vi "Dashboard Main.vi"() -> ()   [LabVIEW 2012]
uses:
  2013ROBOT!/Auto State Selector.ctl
  <vilib>/event_ctls.llb/eventvkey.ctl
  <vilib>/Utility/config.llb/Read Key (String).vi
  <vilib>/Utility/config.llb/Read Key (I32).vi
  <vilib>/Utility/config.llb/Write Key (String).vi
  <vilib>/Utility/config.llb/Write Key (I32).vi
  <vilib>/Utility/config.llb/NI_LVConfig.lvlib
panel:
  out "Bail Climb":bool
  out "Big Hooks on Bar":bool
  out "High gear - Low gear":bool
  out "Shooter Speed (ft/s)":dbl(knob) scale=0.0..400.0
  in  "Auto State Selector":T1
  out "Battery?":u8(slide) scale=0.0..100.0
  out "Tank Pressure (psi)":dbl(knob) scale=0.0..200.0
  out "Compressor":bool
  out "Climbing":bool
  in  "Camera Settings":T2={"Frate Rate"=30, "Compression"=30, "Size"=1} {"Frate Rate" scale=1.0..30.0; "Size" items=["640x480", "320x240", "160x120"]}
  out "Mode":T3(ring)=enum."Auto Disabled"
  out "Camera IP":string
  out "Robot IP":string
  in  "Dashboard Tab":enum32{"Operation", "Test", "Checklist"}(tab)
  in  "Slider":dbl(slide) scale=0.0..100.0 scale format="%#_3g"
  in  "On/Off":bool caption="Solenoid"
  in  "Test Name":u16(ring) items=["Select the test to run...", "Example Test", "-------------------------------", "List of tests is built in robot code.", "Replace with your own automated tests."]
  in  "Test Tree":string(tree)
  in  "Motor":cluster{"Value":dbl, "Enable":bool} {"Value" scale=-1.0..1.0 scale format="%#_3g"}
  out "Progress":T4 {"Test Progress" scale=0.0..100.0}
  in  "Rev/Fwd":cluster{"Forward":bool, "Reverse":bool}
  in  "Ring":u16(ring) items=["Auto", "Fixed indoor", "Fixed outdoor 1", "Fixed outdoor 2", "Fixed fluorescent 1", "Fixed fluorescent 2", "Hold current"]
  in  "Listbox":i32(listbox)
  in  "Viewer":T5(tab)
  out "Mbps":dbl format="%#.1g"
  in  "Enable":bool
  in  "DB Camera Config":bool
  out "Mbps":bool
  out "fps":dbl format="%#.1g"
  out "Image Error Message":string="Timeout in Camera Communications"
  out "Camera Image":T6(plugin-control)
  out "Autolock":bool
  out "Distance from goal (ft)":dbl(slide) scale=0.0..30.0
  out "Buttons 1":cluster{"1":bool, "2":bool, "3":bool}
  out "Kinect 1":cluster{"X":dbl, "Y":dbl, "Z":dbl} {"X" scale=1.0..-1.0; "Y" scale=1.0..-1.0; "Z" scale=1.0..-1.0}
  out "Buttons 2":cluster{"1":bool, "2":bool, "3":bool}
  out "Kinect 2":cluster{"X":dbl, "Y":dbl, "Z":dbl} {"X" scale=1.0..-1.0; "Y" scale=1.0..-1.0; "Z" scale=1.0..-1.0}
  out "Version":string
  out "Skeleton Picture":picture
  out "Players":i8
  out "Tree":string(tree)
  # "Robot IP:"
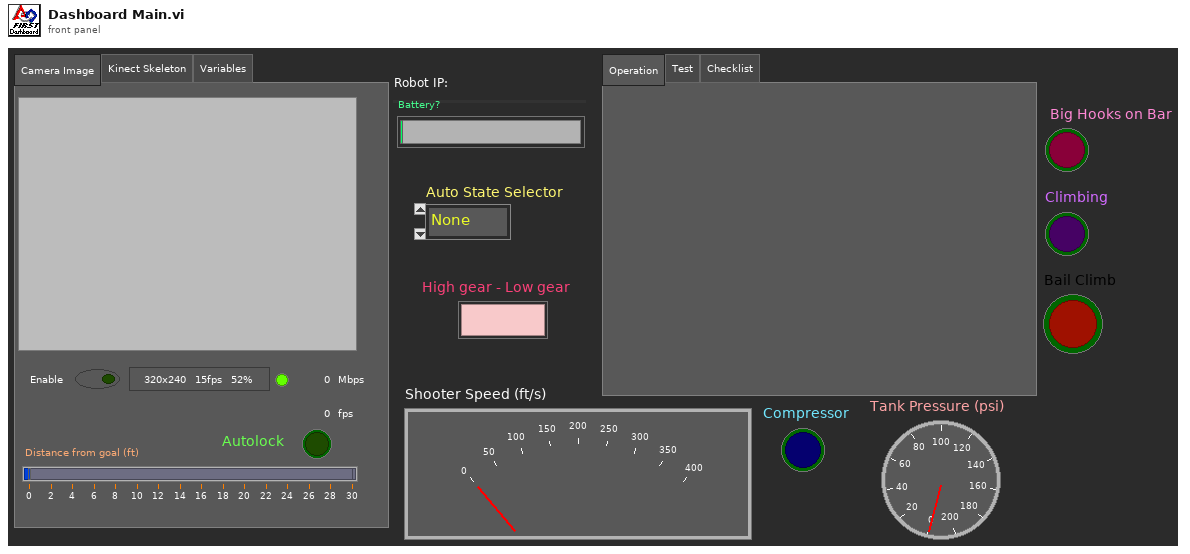
[diagram p1: front panel]
types:
  T1 = typedef "Auto State Selector.ctl" = enum16{"None", "Fire 2x", "Fire 3x", "Dump in low goal"}
  T2 = cluster{"Frate Rate":i32, "Compression":i32, "Size":u16}
  T3 = enum8{"Tele-Op Disabled", "Tele-Op Enabled", "Auto Disabled", "Auto Enabled", "Test Disabled", "Test Enabled", ""}
  T4 = cluster{"Test Progress":u8, "Test Progress Text":string}
  T5 = enum32{"Camera Image", "Kinect Skeleton", "Variables"}
  T6 = typedef "IMAQ Image.ctl" = refnum<image>
  T7 = typedef "Image Type" = u32
  T8 = typedef "LVBoundsTypeDef.ctl" = cluster{"Width":u32, "Height":u32}
  T9 = typedef "SkeletonTrackState.ctl" = enum32{"NotTracked", "PositionOnly", "Tracked"}
  T10 = cluster{"TrackingState":u8[], "Position":cluster{"x":sgl, "y":sgl, "z":sgl}, cluster{"x":sgl, "y":sgl, "z":sgl, sgl}[], "TrackState":T9}
  T11 = cluster{cluster{"ScaledToPercentRange":dbl, "ScaledToPercentRange":dbl, "ScaledToPercentRange":dbl}, cluster{bool, bool, bool}}[]
  T12 = cluster{cluster{"ScaledToPercentRange":dbl, "ScaledToPercentRange":dbl, "ScaledToPercentRange":dbl}, cluster{bool, bool, bool}}
  T13 = cluster{"ScaledToPercentRange":dbl, "ScaledToPercentRange":dbl, "ScaledToPercentRange":dbl}
  T14 = typedef "LVRectTypeDef.ctl" = cluster{"Left":i16, "Top":i16, "Right":i16, "Bottom":i16}
  T15 = cluster{"Competition mode":bool, "Robot Link":bool, "Autonomous":bool, "Enabled":bool, "E-Stop":bool, "Simulated":bool, "TestMode":bool, "Docked Window":bool}
  T16 = typedef "NI_LVConfig.lvlib/Config Data RefNum.ctl" = refnum<k1>
  T17 = typedef "eventvkey.ctl" = enum16{"ASCII", "Enter", "Return", "Shift", "Ctrl", "Alt", "Cmd", "Opt", "Caps", "NumLock", "Clear", "Break", "Up", "Down", "Left", "Right", "Insert", "Delete", "Home", "End", "PageUp", "PageDown", "Escape", "Help", "Pause", "ScrollLock", "F1", "F2", "F3", "F4", "F5", "F6", "F7", "F8", "F9", "F10", "F11", "F12", "F13", "F14", "F15", "F16", "F17", "F18", "F19", "F20", "F21", "F22", "F23", "F24", "Play", "VolumeUp", "VolumeDown", "Mute", "Two Byte Char"}
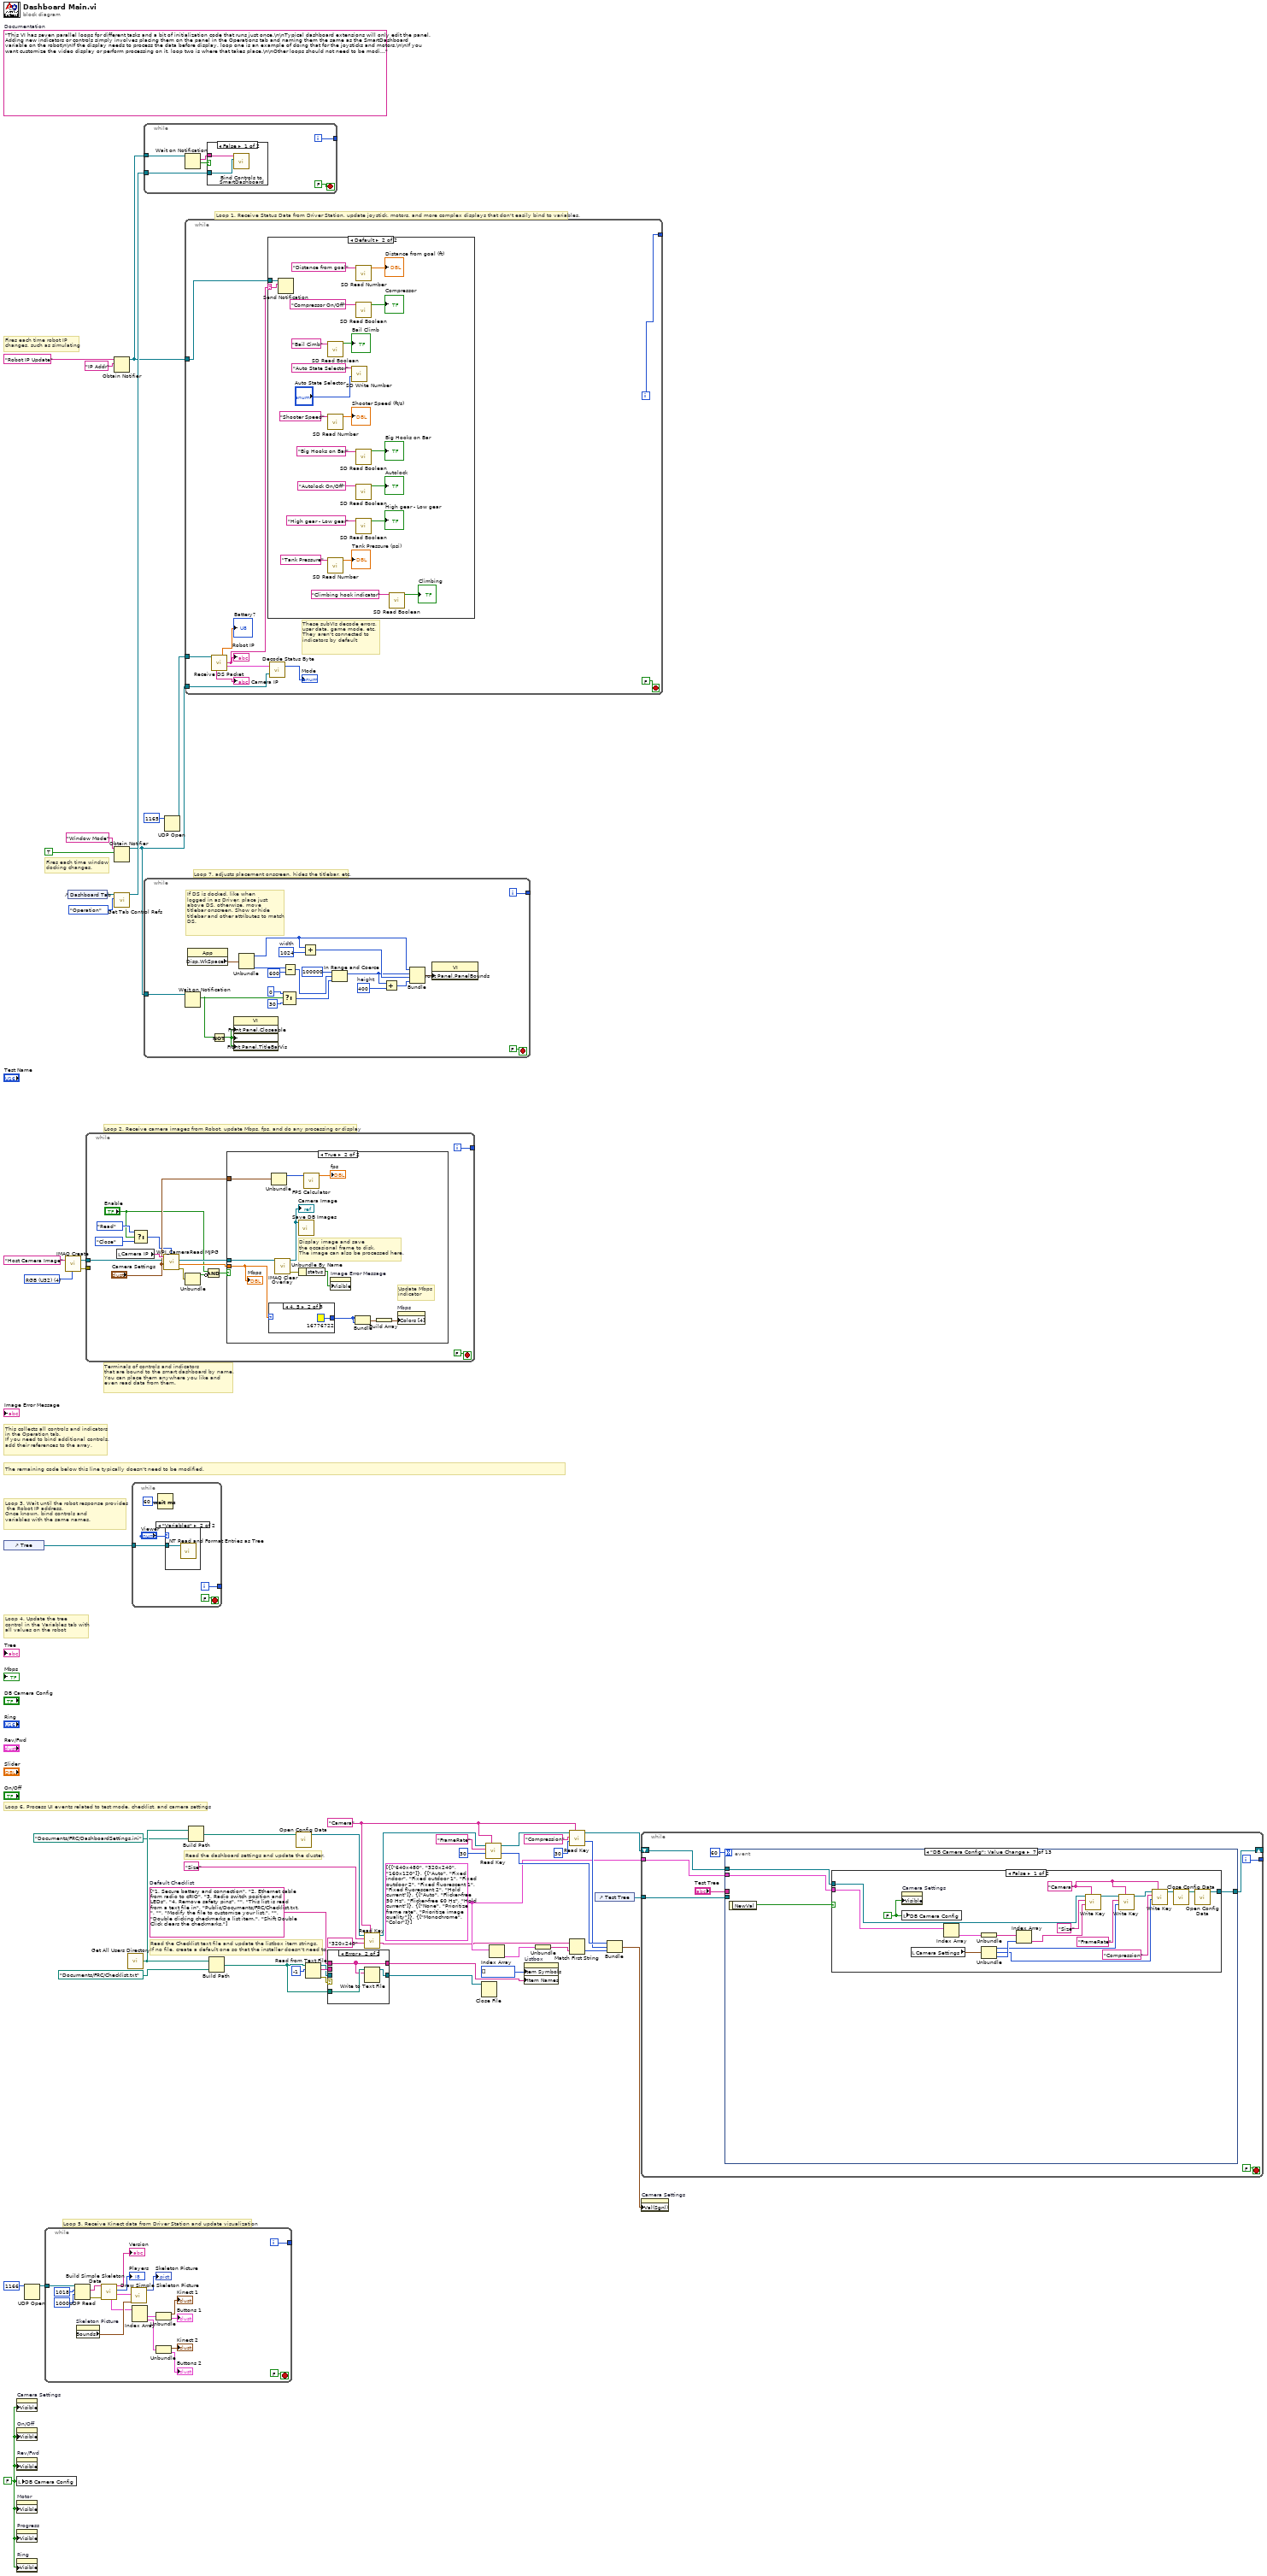
[diagram p0: block diagram]
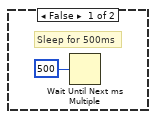
[diagram p3: hidden frame]
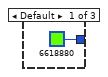
[diagram p4: hidden frame]
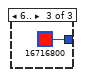
[diagram p5: hidden frame]
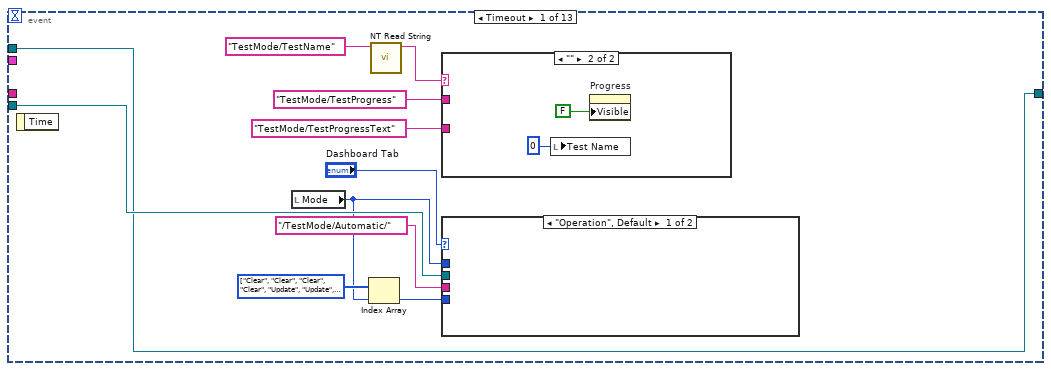
[diagram p7: hidden frame]
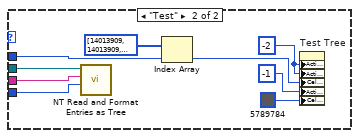
[diagram p8: hidden frame]
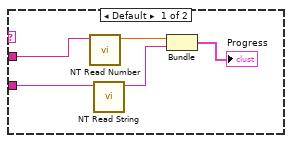
[diagram p9: hidden frame]
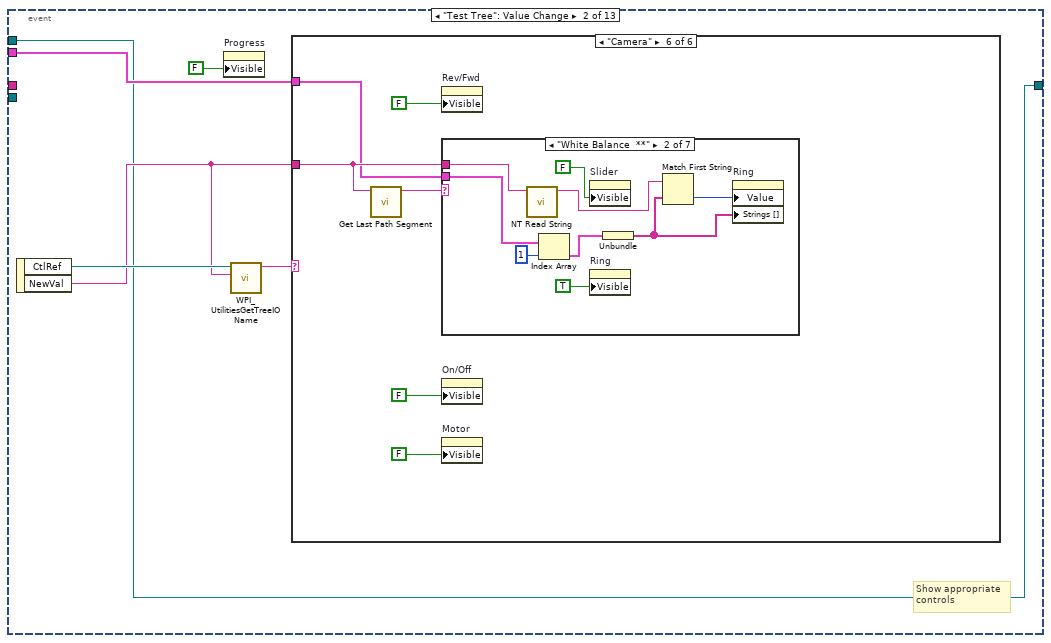
[diagram p10: hidden frame]
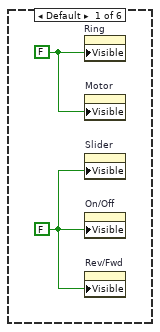
[diagram p11: hidden frame]
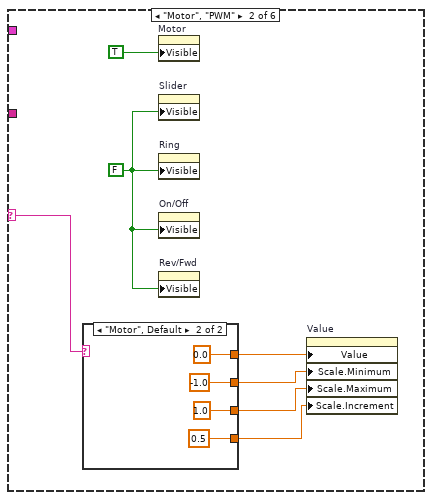
[diagram p12: hidden frame]
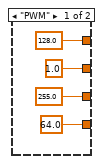
[diagram p13: hidden frame]
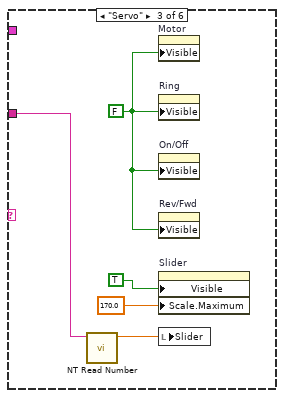
[diagram p14: hidden frame]
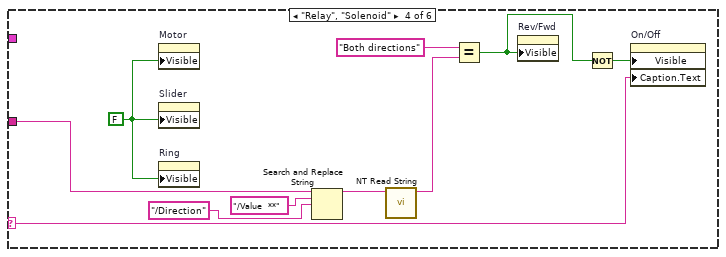
[diagram p15: hidden frame]
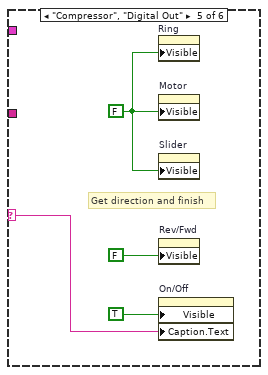
[diagram p16: hidden frame]
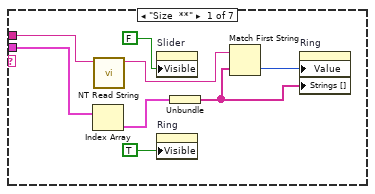
[diagram p17: hidden frame]
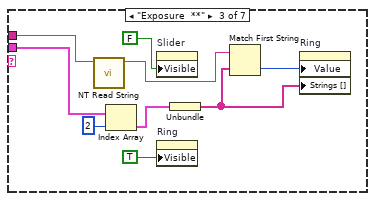
[diagram p18: hidden frame]
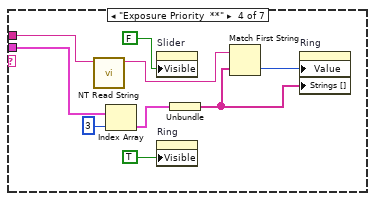
[diagram p19: hidden frame]
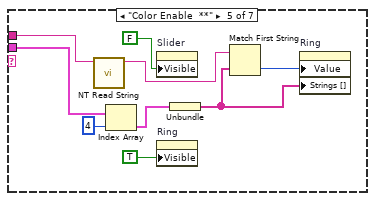
[diagram p20: hidden frame]
diagram:
  w21 = "Camera"
  w13 = cluster{string[]}[] [{["640x480", "320x240", "160x120"]}, {["Auto", "Fixed indoor", "Fixed outdoor 1", "Fixed outdoor 2", "Fixed fluorescent 1", "Fixed fluorescent 2", "Hold current"]}, {["Auto", "Flicker-free 50 Hz", "Flicker-free 60 Hz", "Hold current"]}, {["None", "Prioritize frame rate", "Prioritize image quality"]}, {["Monochrome", "Color"]}]
  w29 = string[] ["1. Secure battery and connection", "2. Ethernet cable from radio to cRIO", "3. Radio switch position and LEDs", "4. Remove safety pins", "", "This list is read from a text file in", "Public/Documents/FRC/Checklist.txt.", "", "Modify the file to customize your list.", "", "Double clicking checkmarks a list item.", "Shift Double Click clears the checkmarks."]  # Default Checklist
  w27 = FALSE ("Visible")
  (unwired) "This VI has seven parallel loops for different tasks and a bit of initialization code that runs just once.\n\nTypical dashboard extensions will only edit the panel. Adding new indicators or controls simply involves placing them on the panel in the Operations tab and naming them the same as the SmartDashboard variable on the robot\n\nIf the display needs to process the data before display, loop one is an example of doing that for the joysticks and motors.\n\nIf you want customize the video display or perform processing on it, loop two is where that takes place.\n\nOther loops should not need to be modified. They are pretty standard, and document the task they perform."  # Documentation
  w50 = T7 4 items=["Grayscale (U8)", "Grayscale (I16)", "Grayscale (SGL)", "Complex (CSG)", "RGB (U32)", "HSL (U32)", "RGB (U64)"] ("Image Type")
  # "Fires each time robot IP\nchanges, such as simulating"
  # "Fires each time window\ndocking changes."
  # "Read the Checklist text file and update the listbox item strings.\nIf no file, create a default one so that the installer doesn't need to."
  # "This collects all controls and indicators\nin the Operation tab.\nIf you need to bind additional controls,\nadd their references to the array."
  # "The remaining code below this line typically doesn't need to be modified."
  # "Loop 6. Process UI events related to test mode, checklist, and camera settings"
  # "Read the dashboard settings and update the cluster."
  # "Terminals of controls and indicators\nthat are bound to the smart dashboard by name.\nYou can place them anywhere you like and\neven read data from them."
  # "Loop 4. Update the tree\ncontrol in the Variables tab with\nall values on the robot"
  # "Loop 3. Wait until the robot response provides\n the Robot IP address.\nOnce known, bind controls and\nvariables with the same names."
  # "Loop 5. Receive Kinect data from Driver Station and update visualization"
  # "Loop 7. adjusts placement onscreen, hides the titlebar, etc."
  # "Loop 1. Receive Status Data from Driver Station, update joystick, motors, and more complex displays that don't easily bind to variables."
  # "Loop 2. Receive camera images from Robot, update Mbps, fps, and do any processing or display"
  n1 = control-ref of="Tree"() -> (w2:refnum<vi>)
  n2 = property on="Camera Settings" class="Clust (strict)"("Visible"=w27) -> ()  [unwired: 2 in, 2 out]
  n3 = property on="On/Off" class="Bool (strict)"("Visible"=w27) -> ()  [unwired: 2 in, 2 out]
  n4 = property on="Rev/Fwd" class="Clust (strict)"("Visible"=w27) -> ()  [unwired: 2 in, 2 out]
  n5 = local write "DB Camera Config"(w27) -> ()
  n6 = property on="Motor" class="Clust (strict)"("Visible"=w27) -> ()  [unwired: 2 in, 2 out]
  n7 = property on="Progress" class="Clust (strict)"("Visible"=w27) -> ()  [unwired: 2 in, 2 out]
  n8 = property on="Ring" class="Ring (strict)"("Visible"=w27) -> ()  [unwired: 2 in, 2 out]
  n9 = UDP Open(11:u16 1166 ("port")) -> (port=w45:refnum<k16>)  [unwired: 2 in, 4 out]
  n10 = while {
    tunnel: w45 -> [w69]
    tunnel: [w54] -> _
    i -> [w54]
    stop <- FALSE stop-if-true
    n11 = UDP Read(connection ID=w69, max size (548)=1018 ("bytes to read"), timeout ms (25000)=1000) -> (data out=w63:string, error out=w53:errorcluster)  [unwired: 1 in, 3 out]
    n12 = property on="Skeleton Picture" class="Pict"() -> ("Bounds"=w65:T8)  [unwired: 2 in, 2 out]
    n13 = call "Build Simple Skeleton Data.vi"("error in (no error)"=w53, "data in"=w63) -> ("Skeleton Data"=w64:T10, "NumPlayers"=→"Players":i8, "Version String"=→"Version":string, "Simple Joystick Info"=w61:T11)  [unwired: 5 in, 1 out]
    n14 = call "Draw Simple Skeleton Picture.vi"("Bounds"=w65, "Simple Skeleton"=w64) -> ("new picture out"=→"Skeleton Picture":picture)  [unwired: 9 in]
    n15 = Index Array(array=w61) -> (element #1=w60:T12, element #2=w59:T12)  [unwired: 2 in]
    n16 = Unbundle(w60) -> (→"Kinect 1":T13, →"Buttons 1":cluster{bool, bool, bool})
    n17 = Unbundle(w59) -> (→"Kinect 2":T13, →"Buttons 2":cluster{bool, bool, bool})
  }
  n18 = call "IMAQ Create"("Image Name"="Host Camera Image", "Image Type"=w50) -> ("New Image"=w48:T6, "error out"=w47:errorcluster)  [unwired: 2 in, 1 out]
  n19 = control-ref of="Dashboard Tab"() -> (w43:refnum<vi>)
  n20 = while {
    tunnel: w48 -> [w81]
    tunnel: w47 -> [_]
    tunnel: [w84] -> _
    i -> [w84]
    stop <- FALSE stop-if-true
    n21 = local read "Camera IP"() -> (w83:string)
    n22 = Select(t=enum16{"Read", "Reopen", "Close"}."Read" ("Operation"), s="Enable", f=enum16{"Read", "Reopen", "Close"}."Close" ("Operation")) -> (s? t:f=w76:enum16{"Read", "Reopen", "Close"})
    n23 = call <vilib>:"WPI_CameraRead MJPG.vi"("Operation"=w76, "Camera Settings"="Camera Settings", "Image"=w81, "address"=w83) -> ("error out"=w75:errorcluster, "Bandwidth (kbps)"=w79:dbl, "Image Out"=w80:T6)  [unwired: 5 in]
    n24 = Unbundle(w75) -> ("status"=w73:bool)  [unwired: 2 out]
    n25 = Compound Arithmetic op=AND("Enable", invert w73) -> (w72:bool)
    n26 = case shown="True" w72 {
      tunnel: "Camera Settings" -> [_ w88]
      tunnel: w80 -> [_ w91]
      tunnel: w79 -> [_ w90]
      frame False {
        # "Sleep for 500ms"
        n27 = Wait Until Next ms Multiple(millisecond multiple=u32 500) -> ()  [unwired: 1 out]
      }
      frame True {
        # "Display image and save\nthe occasional frame to disk.\nThe image can also be processed here."
        # "Update Mbps\nindicator"
        n28 = case shown="4, 5" w90 {
          tunnel: [u32 6618880 ("Color Box") u32 16776722 ("Color Box") u32 16716800 ("Color Box")] -> w92
          frame Default {
          }
          frame 4, 5 {
          }
          frame 6.. {
          }
        }
        n29 = Unbundle(w88) -> ("Frate Rate"=w87:i32)  [unwired: 2 out]
        n30 = call "IMAQ Clear Overlay"("Image"=w91) -> ("error out"=w96:errorcluster, "Image Out"=w95:T6)  [unwired: 2 in, 7 out]
        "Camera Image" <- w95
        n31 = call "Save DB Images.vi"("Image"=w95) -> ()  [unwired: 2 in, 1 out]
        n32 = Unbundle By Name(w96) -> ("status"=w97:bool)
        n33 = call "FPS Calculator.vi"("Average Count"=w87) -> ("fps"=→"fps":dbl)  [unwired: 10 in]
        n34 = property on="Image Error Message" class="Str"("Visible"=w97) -> ()  [unwired: 2 in, 2 out]
        n35 = Bundle("Color Box"=w92, "Color Box"=w92) -> (w94:cluster{"Color Box":u32, "Color Box":u32})  [unwired: 1 out]
        n36 = Build Array(w94) -> (w93:cluster{"Color Box":u32, "Color Box":u32}[])
        n37 = property on="Mbps" class="Bool (strict)"("Colors [4]"=w93) -> ()  [unwired: 2 in, 2 out]
        "Mbps" <- w90
      }
    }
  }
  n38 = Obtain Notifier(name (unnamed)="Robot IP Update", notification data type="IP Addr" ("name (unnamed)")) -> (notifier out=w40:refnum<notifier>)  [unwired: 2 in, 2 out]
  n39 = Obtain Notifier(name (unnamed)="Window Mode", notification data type=TRUE) -> (notifier out=w33:refnum<notifier>)  [unwired: 2 in, 2 out]
  n40 = call <vilib>:"Get Tab Control Refs.vi"("Page Index"=enum32{"Operation", "Test"}."Operation" ("Dashboard Tab"), "TabControl in"=w43) -> ("ControlsOnPage"=w44:refnum<vi>[])  [unwired: 9 in]
  n41 = call "Get All Users Directory.vi"() -> ("All User Path"=w26:path)
  n42 = while {
    tunnel: [w102] -> _
    tunnel: w2 -> [w101]
    i -> [w102]
    stop <- FALSE stop-if-true
    n43 = Wait (ms)(milliseconds to wait=u32 60) -> ()  [unwired: 1 out]
    n44 = case shown="\"Variables\"" "Viewer" {
      tunnel: w101 -> [_ w106]
      frame Default {
      }
      frame "Variables" {
        n45 = call <vilib>:"NT Read and Format Entries as Tree.vi"("Tree Refnum"=w106) -> ()  [unwired: 9 in, 2 out]
      }
    }
  }
  n46 = while {
    tunnel: w44 -> [w112]
    tunnel: w40 -> [w109]
    tunnel: [w107] -> _
    i -> [w107]
    stop <- FALSE stop-if-true
    n47 = Wait on Notification(notifier=w109) -> (notification=w108:string, timed out?=w110:bool)  [unwired: 3 in, 2 out]
    n48 = case shown="False" w110 {
      tunnel: w112 -> [w114 _]
      tunnel: w108 -> [w113 _]
      frame False {
        n49 = call <vilib>:"Bind Controls to SmartDashboard.vi"("Bound Control Refs"=w114, "Server IP Address"=w113) -> ()  [unwired: 10 in]
      }
      frame True {
      }
    }
  }
  n50 = while {
    tunnel: w33 -> [w133]
    tunnel: [w131] -> _
    i -> [w131]
    stop <- FALSE stop-if-true
    w123 = 1024  # width
    w126 = 400  # height
    # "If DS is docked, like when\nlogged in as Driver, place just\nabove DS, otherwise, move\ntitlebar onscreen. Show or hide\ntitlebar and other attributes to match\nDS."
    n51 = Wait on Notification(notifier=w133) -> (notification=w118:bool)  [unwired: 3 in, 3 out]
    n52 = property class="App"() -> ("Disp.WkSpace"=w129:T14)  [unwired: 2 in, 2 out]
    n53 = Not(x=w118) -> (.not. x?=w132:bool)
    n54 = property class="VI"("Front Panel.Closeable"=w132, "Front Panel.Minimizeable"=w132, "Front Panel.TitleBarVis"=w132) -> ()  [unwired: 2 in, 2 out]
    n55 = Unbundle(w129) -> ("Left"=w127:i16, "Bottom"=w124:i16)  [unwired: 2 out]
    n56 = Select(t=0, s=w118, f=30) -> (s? t:f=w117:i32)
    n57 = Subtract(x=w124, y=600) -> (x-y=w121:i32)
    n58 = Add(x=w127, y=w123) -> (x+y=w128:i32)
    n59 = In Range and Coerce(upper limit=100000, x=w121, lower limit=w117) -> (coerced(x)=w115:i32)  [unwired: 1 out]
    n60 = Add(x=w115, y=w126) -> (x+y=w125:i32)
    n61 = Bundle("Left"=w127, w115, w128, w125) -> (w130:cluster{"Left":i16, i32, i32, i32})  [unwired: 1 out]
    n62 = property class="VI"("Front Panel.PanelBounds"=w130) -> ()  [unwired: 2 in, 2 out]
  }
  n63 = UDP Open(11:u16 1165 ("port")) -> (port=w51:refnum<k16>)  [unwired: 2 in, 4 out]
  n64 = while {
    tunnel: w51 -> [w142]
    tunnel: w40 -> [w137]
    tunnel: w33 -> [w141]
    tunnel: [w138] -> _
    i -> [w138]
    stop <- FALSE stop-if-true
    # "These subVIs decode errors, user data, game mode, etc.\nThey aren't connected to indicators by default"
    n65 = call "Receive DS Packet.vi"("Recv Socket"=w142) -> ("Battery"=→"Battery?":sgl, "Robot IP Address"=w136:string, "Status"=w143:T15, "Camera IP Address"=→"Camera IP":string)  [unwired: 1 in, 10 out]
    "Robot IP" <- w136
    n66 = case shown="Default" w136 {
      selector: w136 -> [_ w165]
      tunnel: w137 -> [_ w166]
      frame "0.0.0.0" {
        # "Robot not responding, don't poll the variables"
      }
      frame Default {
        n67 = Send Notification(notification=w165, notifier=w166) -> ()  [unwired: 1 in, 2 out]
        n68 = call <vilib>:"SD Read Boolean.vi"("Name"="Bail Cimb") -> ("Boolean"=→"Bail Climb":bool)  [unwired: 8 in, 2 out]
        n69 = call <vilib>:"SD Read Number.vi"("Name"="Shooter Speed") -> ("Numeric"=→"Shooter Speed (ft/s)":dbl)  [unwired: 8 in, 2 out]
        n70 = call <vilib>:"SD Read Number.vi"("Name"="Tank Pressure") -> ("Numeric"=→"Tank Pressure (psi)":dbl)  [unwired: 8 in, 2 out]
        n71 = call <vilib>:"SD Write Number.vi"("Numeric"="Auto State Selector", "Name"="Auto State Selector") -> ()  [unwired: 8 in, 2 out]
        n72 = call <vilib>:"SD Read Number.vi"("Name"="Distance from goal") -> ("Numeric"=→"Distance from goal (ft)":dbl)  [unwired: 8 in, 2 out]
        n73 = call <vilib>:"SD Read Boolean.vi"("Name"="Compressor On/Off") -> ("Boolean"=→"Compressor":bool)  [unwired: 8 in, 2 out]
        n74 = call <vilib>:"SD Read Boolean.vi"("Name"="Big Hooks on Bar") -> ("Boolean"=→"Big Hooks on Bar":bool)  [unwired: 8 in, 2 out]
        n75 = call <vilib>:"SD Read Boolean.vi"("Name"="Autolock On/Off") -> ("Boolean"=→"Autolock":bool)  [unwired: 8 in, 2 out]
        n76 = call <vilib>:"SD Read Boolean.vi"("Name"="High gear - Low gear") -> ("Boolean"=→"High gear - Low gear":bool)  [unwired: 8 in, 2 out]
        n77 = call <vilib>:"SD Read Boolean.vi"("Name"="Climbing hook indicator") -> ("Boolean"=→"Climbing":bool)  [unwired: 8 in, 2 out]
      }
    }
    n78 = call "Decode Status Byte.vi"("Window Mode Notifier"=w141, "Status"=w143) -> ("Mode"=→"Mode":T3)  [unwired: 1 out]
  }
  n79 = Build Path(base path=w26, name or relative path=path "Documents/FRC/DashboardSettings.ini") -> (appended path=w25:path)
  n80 = Build Path(base path=w26, name or relative path=path "Documents/FRC/Checklist.txt") -> (appended path=w30:path)
  n81 = call <vilib>:"Open Config Data.vi"("configuration file path"=w25) -> ("refnum"=w24:T16)  [unwired: 8 in, 2 out]
  n82 = Read from Text File(file (use dialog)=w30, count=-1 ("timeout ms (25000)")) -> (refnum out=w8:refnum<file>, text=w31:string[], error out=w32:errorcluster)  [unwired: 2 in, 1 out]
  n83 = case shown="Error" w32 {
    tunnel: w31 -> [w168 _]
    tunnel: [w168 w170] -> w28
    tunnel: w29 -> [_ w170]
    tunnel: w30 -> [_ w171]
    tunnel: [w167 w169] -> w7
    tunnel: w8 -> [w167 _]
    frame No Error {
    }
    frame Error {
      n84 = Write to Text File(file (use dialog)=w171, text=w170) -> (refnum out=w169:refnum<file>)  [unwired: 2 in, 2 out]
    }
  }
  n85 = call-poly <vilib>:"Read Key.vi"("section"=w21, "default value"="320x240", "key"="Size", "refnum"=w24) -> ("value"=w11:string, "refnum out"=w6:T16)  [unwired: 2 in, 4 out]
  n86 = Close File(refnum=w7) -> ()  [unwired: 1 in, 2 out]
  n87 = call-poly <vilib>:"Read Key.vi"("section"=w21, "default value"=30, "key"="FrameRate", "refnum"=w6) -> ("value"=w16:i32, "refnum out"=w5:T16)  [unwired: 1 in, 5 out]
  n88 = Index Array(array=w13) -> (element=w14:cluster{string[]})  [unwired: 1 in]
  n89 = property on="Listbox" class="LstBox (strict)"("Item Symbols"=i32[] [], "Item Names"=w28) -> ()  [unwired: 2 in, 2 out]
  n90 = Unbundle(w14) -> (w12:string[])
  n91 = call-poly <vilib>:"Read Key.vi"("section"=w21, "default value"=30, "key"="Compression", "refnum"=w5) -> ("value"=w15:i32, "refnum out"=w3:T16)  [unwired: 1 in, 5 out]
  n92 = Match First String(2:w12, 3:w11) -> (0:w10:i32)  [unwired: 1 out]
  n93 = control-ref of="Test Tree"() -> (w1:refnum<vi>)
  n94 = Bundle("value"=w16, "value"=w15, "index"=w10) -> (w4:cluster{"value":i32, "value":i32, "index":i32})  [unwired: 1 out]
  n95 = while {
    tunnel: w13 -> [w176]
    shift-right: [w175] -> _
    shift-left: w3 -> [w174]
    tunnel: [w173] -> _
    tunnel: w1 -> [w172]
    i -> [w173]
    stop <- FALSE stop-if-true
    n96 = event shown="[6] \"DB Camera Config\": Value Change" {
      selector: _ -> [_ _ _ _ _ _ _ _ _ _ _ _ _]
      dyn-events: _ -> [_ _ _ _ _ _ _ _ _ _ _ _ _]
      timeout: u32 60 ("milliseconds to wait") -> [_ _ _ _ _ _ _ _ _ _ _ _ _]
      tunnel: w172 -> [w186 _ _ _ _ _ _ _ _ _ _ _ _]
      tunnel: "Test Tree" -> [_ _ _ _ _ _ _ _ w380 w388 w390 w394 w402]
      tunnel: w176 -> [_ w208 _ _ _ _ w344 w374 _ _ _ _ _]
      tunnel: [w180 w207 _ w310 w318 w330 w343 w367 w379 w386 w389 w393 w401] -> w175
      tunnel: w174 -> [w180 w207 _ w310 w318 w330 w342 w367 w379 w386 w389 w393 w401]
      event Timeout {
        w185 = enum16{"Update", "Clear"}[] [enum."Clear", enum."Clear", enum."Clear", enum."Clear", enum."Update", enum."Update", enum."Clear"] items=["Update", "Clear"]
        n97 = event-data() -> ()  [unwired: 1 in, 1 out]
        n98 = local read "Mode"() -> (w183:T3)
        n99 = Index Array(array=w185, index=w183) -> (element=w184:enum16{"Update", "Clear"})
        n100 = call <vilib>:"NT Read String.vi"("Name"="TestMode/TestName") -> ("String"=w189:string)  [unwired: 9 in, 1 out]
        n101 = case shown="\"\"" w189 {
          tunnel: "TestMode/TestProgress" ("Name") -> [w201 _]
          tunnel: "TestMode/TestProgressText" ("Name") -> [w200 _]
          frame Default {
            n102 = call <vilib>:"NT Read Number.vi"("Name"=w201) -> ("Numeric"=w202:dbl)  [unwired: 9 in, 1 out]
            n103 = call <vilib>:"NT Read String.vi"("Name"=w200) -> ("String"=w203:string)  [unwired: 9 in, 1 out]
            n104 = Bundle("Numeric"=w202, "String"=w203) -> (→"Progress":cluster{"Numeric":dbl, "String":string})  [unwired: 1 in]
          }
          frame "" {
            n105 = local write "Test Name"(u16 0) -> ()
            n106 = property on="Progress" class="Clust (strict)"("Visible"=FALSE) -> ()  [unwired: 2 in, 2 out]
          }
        }
        n107 = case shown="\"Operation\", Default" "Dashboard Tab" {
          tunnel: w186 -> [_ w199]
          tunnel: "/TestMode/Automatic/" ("Name Pattern") -> [_ w198]
          tunnel: w184 -> [_ w197]
          tunnel: w183 -> [_ w195]
          frame "Operation", Default {
          }
          frame "Test" {
            w194 = -2 ("Active Item:Row Number")
            n108 = call <vilib>:"NT Read and Format Entries as Tree.vi"("Operation"=w197, "Name Pattern"=w198, "Tree Refnum"=w199) -> ()  [unwired: 7 in, 2 out]
            n109 = Index Array(array=u32[] [14013909, 14013909, 14013909, 14013909, 14013909, 16777215, 14013909], index=w195) -> (element=w193:u32)
            n110 = property on="Test Tree" class="Tree (strict)"("Active Item Row Number"=w194, "ActiveColNum"=w194, "CellBG"=w193, "Active Item Row Number"=-1 ("Active Item:Row Number"), "CellBG"=u32 5789784 ("Color Box")) -> ()  [unwired: 2 in, 2 out]
          }
        }
      }
      event "Test Tree": Value Change {
        # "Show appropriate\ncontrols"
        n111 = event-data() -> ("CtlRef"=w211:refnum<vi>, "NewVal"=w209:string)  [unwired: 1 in]
        n112 = property on="Progress" class="Clust (strict)"("Visible"=FALSE) -> ()  [unwired: 2 in, 2 out]
        n113 = call <vilib>:"WPI_UtilitiesGetTreeIOName.vi"("NewVal"=w209, "TreeControl in"=w211) -> ("I/O Name"=w212:string)  [unwired: 9 in]
        n114 = case shown="\"Camera\"" w212 {
          selector: w212 -> [_ w219 _ w237 w246 _]
          tunnel: w209 -> [_ _ w234 w236 _ w253]
          tunnel: w208 -> [_ _ _ _ _ w252]
          frame Default {
            w214 = FALSE ("Visible")
            w213 = FALSE ("Visible")
            n115 = property on="Ring" class="Ring (strict)"("Visible"=w213) -> ()  [unwired: 2 in, 2 out]
            n116 = property on="Motor" class="Clust (strict)"("Visible"=w213) -> ()  [unwired: 2 in, 2 out]
            n117 = property on="Slider" class="Slide (strict)"("Visible"=w214) -> ()  [unwired: 2 in, 2 out]
            n118 = property on="On/Off" class="Bool (strict)"("Visible"=w214) -> ()  [unwired: 2 in, 2 out]
            n119 = property on="Rev/Fwd" class="Clust (strict)"("Visible"=w214) -> ()  [unwired: 2 in, 2 out]
          }
          frame "Motor", "PWM" {
            w220 = FALSE ("Visible")
            n120 = case shown="\"Motor\", Default" w219 {
              tunnel: [1.0 ("Value") -1.0 ("Value")] -> w218
              tunnel: [255.0 ("Value") 1.0 ("Value")] -> w217
              tunnel: [128.0 ("Value") 0.0 ("Value")] -> w216
              tunnel: [64.0 ("Value") 0.5 ("Value")] -> w215
              frame "PWM" {
              }
              frame "Motor", Default {
              }
            }
            n121 = property on="Motor" class="Clust (strict)"("Visible"=TRUE) -> ()  [unwired: 2 in, 2 out]
            n122 = property on="Slider" class="Slide (strict)"("Visible"=w220) -> ()  [unwired: 2 in, 2 out]
            n123 = property on="Ring" class="Ring (strict)"("Visible"=w220) -> ()  [unwired: 2 in, 2 out]
            n124 = property on="On/Off" class="Bool (strict)"("Visible"=w220) -> ()  [unwired: 2 in, 2 out]
            n125 = property on="Rev/Fwd" class="Clust (strict)"("Visible"=w220) -> ()  [unwired: 2 in, 2 out]
            n126 = property on="Value" class="Slide (strict)"("Value"=w216, "Scale.Minimum"=w218, "Scale.Maximum"=w217, "Scale.Increment"=w215) -> ()  [unwired: 2 in, 2 out]
          }
          frame "Servo" {
            w232 = FALSE ("Visible")
            n127 = call <vilib>:"NT Read Number.vi"("Name"=w234) -> ("Numeric"=w233:dbl)  [unwired: 9 in, 1 out]
            n128 = property on="Motor" class="Clust (strict)"("Visible"=w232) -> ()  [unwired: 2 in, 2 out]
            n129 = property on="Ring" class="Ring (strict)"("Visible"=w232) -> ()  [unwired: 2 in, 2 out]
            n130 = property on="On/Off" class="Bool (strict)"("Visible"=w232) -> ()  [unwired: 2 in, 2 out]
            n131 = property on="Rev/Fwd" class="Clust (strict)"("Visible"=w232) -> ()  [unwired: 2 in, 2 out]
            n132 = property on="Slider" class="Slide (strict)"("Visible"=TRUE, "Scale.Maximum"=170.0 ("Scale.Range:Maximum")) -> ()  [unwired: 2 in, 2 out]
            n133 = local write "Slider"(w233) -> ()
          }
          frame "Relay", "Solenoid" {
            w235 = FALSE ("Visible")
            n134 = property on="Motor" class="Clust (strict)"("Visible"=w235) -> ()  [unwired: 2 in, 2 out]
            n135 = property on="Slider" class="Slide (strict)"("Visible"=w235) -> ()  [unwired: 2 in, 2 out]
            n136 = property on="Ring" class="Ring (strict)"("Visible"=w235) -> ()  [unwired: 2 in, 2 out]
            n137 = Search and Replace String(input string=w236, search string="/Value  **", replace string="/Direction") -> (result string=w242:string)  [unwired: 5 in, 3 out]
            n138 = call <vilib>:"NT Read String.vi"("Name"=w242) -> ("String"=w240:string)  [unwired: 9 in, 1 out]
            n139 = Equal?(x="Both directions", y=w240) -> (x = y?=w238:bool)
            n140 = property on="Rev/Fwd" class="Clust (strict)"("Visible"=w238) -> ()  [unwired: 2 in, 2 out]
            n141 = Not(x=w238) -> (.not. x?=w239:bool)
            n142 = property on="On/Off" class="Bool (strict)"("Visible"=w239, "Caption.Text"=w237) -> ()  [unwired: 2 in, 2 out]
          }
          frame "Compressor", "Digital Out" {
            w245 = FALSE ("Visible")
            # "Get direction and finish"
            n143 = property on="Ring" class="Ring (strict)"("Visible"=w245) -> ()  [unwired: 2 in, 2 out]
            n144 = property on="Motor" class="Clust (strict)"("Visible"=w245) -> ()  [unwired: 2 in, 2 out]
            n145 = property on="Slider" class="Slide (strict)"("Visible"=w245) -> ()  [unwired: 2 in, 2 out]
            n146 = property on="Rev/Fwd" class="Clust (strict)"("Visible"=FALSE) -> ()  [unwired: 2 in, 2 out]
            n147 = property on="On/Off" class="Bool (strict)"("Visible"=TRUE, "Caption.Text"=w246) -> ()  [unwired: 2 in, 2 out]
          }
          frame "Camera" {
            n148 = call <vilib>:"Get Last Path Segment.vi"("String in"=w253) -> ("String out"=w254:string)  [unwired: 10 in]
            n149 = property on="Rev/Fwd" class="Clust (strict)"("Visible"=FALSE) -> ()  [unwired: 2 in, 2 out]
            n150 = case shown="\"White Balance  **\"" w254 {
              tunnel: w253 -> [w260 w269 w278 w287 w296 _ w302]
              tunnel: w252 -> [w258 w266 w275 w284 w293 _ _]
              frame "Size  **" {
                n151 = Index Array(array=w258) -> (element=w257:cluster{string[]})  [unwired: 1 in]
                n152 = call <vilib>:"NT Read String.vi"("Name"=w260) -> ("String"=w259:string)  [unwired: 9 in, 1 out]
                n153 = property on="Slider" class="Slide (strict)"("Visible"=FALSE) -> ()  [unwired: 2 in, 2 out]
                n154 = property on="Ring" class="Ring (strict)"("Visible"=TRUE) -> ()  [unwired: 2 in, 2 out]
                n155 = Unbundle(w257) -> (w255:string[])
                n156 = Match First String(2:w255, 3:w259) -> (0:w256:i32)  [unwired: 1 out]
                n157 = property on="Ring" class="Ring (strict)"("Value"=w256, "Strings []"=w255) -> ()  [unwired: 2 in, 2 out]
              }
              frame "White Balance  **" {
                n158 = call <vilib>:"NT Read String.vi"("Name"=w269) -> ("String"=w268:string)  [unwired: 9 in, 1 out]
                n159 = Index Array(array=w266, index=1) -> (element=w267:cluster{string[]})
                n160 = property on="Slider" class="Slide (strict)"("Visible"=FALSE) -> ()  [unwired: 2 in, 2 out]
                n161 = property on="Ring" class="Ring (strict)"("Visible"=TRUE) -> ()  [unwired: 2 in, 2 out]
                n162 = Unbundle(w267) -> (w264:string[])
                n163 = Match First String(2:w264, 3:w268) -> (0:w263:i32)  [unwired: 1 out]
                n164 = property on="Ring" class="Ring (strict)"("Value"=w263, "Strings []"=w264) -> ()  [unwired: 2 in, 2 out]
              }
              frame "Exposure  **" {
                n165 = call <vilib>:"NT Read String.vi"("Name"=w278) -> ("String"=w277:string)  [unwired: 9 in, 1 out]
                n166 = Index Array(array=w275, index=2) -> (element=w276:cluster{string[]})
                n167 = property on="Slider" class="Slide (strict)"("Visible"=FALSE) -> ()  [unwired: 2 in, 2 out]
                n168 = property on="Ring" class="Ring (strict)"("Visible"=TRUE) -> ()  [unwired: 2 in, 2 out]
                n169 = Unbundle(w276) -> (w272:string[])
                n170 = Match First String(2:w272, 3:w277) -> (0:w273:i32)  [unwired: 1 out]
                n171 = property on="Ring" class="Ring (strict)"("Value"=w273, "Strings []"=w272) -> ()  [unwired: 2 in, 2 out]
              }
              frame "Exposure Priority  **" {
                n172 = call <vilib>:"NT Read String.vi"("Name"=w287) -> ("String"=w286:string)  [unwired: 9 in, 1 out]
                n173 = Index Array(array=w284, index=3) -> (element=w285:cluster{string[]})
                n174 = property on="Slider" class="Slide (strict)"("Visible"=FALSE) -> ()  [unwired: 2 in, 2 out]
                n175 = property on="Ring" class="Ring (strict)"("Visible"=TRUE) -> ()  [unwired: 2 in, 2 out]
                n176 = Unbundle(w285) -> (w281:string[])
                n177 = Match First String(2:w281, 3:w286) -> (0:w282:i32)  [unwired: 1 out]
                n178 = property on="Ring" class="Ring (strict)"("Value"=w282, "Strings []"=w281) -> ()  [unwired: 2 in, 2 out]
              }
              frame "Color Enable  **" {
                n179 = call <vilib>:"NT Read String.vi"("Name"=w296) -> ("String"=w295:string)  [unwired: 9 in, 1 out]
                n180 = Index Array(array=w293, index=4) -> (element=w294:cluster{string[]})
                n181 = property on="Slider" class="Slide (strict)"("Visible"=FALSE) -> ()  [unwired: 2 in, 2 out]
                n182 = property on="Ring" class="Ring (strict)"("Visible"=TRUE) -> ()  [unwired: 2 in, 2 out]
                n183 = Unbundle(w294) -> (w290:string[])
                n184 = Match First String(2:w290, 3:w295) -> (0:w291:i32)  [unwired: 1 out]
                n185 = property on="Ring" class="Ring (strict)"("Value"=w291, "Strings []"=w290) -> ()  [unwired: 2 in, 2 out]
              }
              frame Default {
                n186 = property on="Slider" class="Slide (strict)"("Visible"=FALSE) -> ()  [unwired: 2 in, 2 out]
                n187 = property on="Ring" class="Ring (strict)"("Visible"=FALSE) -> ()  [unwired: 2 in, 2 out]
              }
              frame "Brightness  **", "Color Level  **", "Compression  **", "FPS  **", "Sharpness  **" {
                n188 = call <vilib>:"NT Read Number.vi"("Name"=w302) -> ("Numeric"=w301:dbl)  [unwired: 9 in, 1 out]
                n189 = property on="Ring" class="Ring (strict)"("Visible"=FALSE) -> ()  [unwired: 2 in, 2 out]
                n190 = property on="Slider" class="Slide (strict)"("Visible"=TRUE, "Scale.Maximum"=100.0 ("Scale.Range:Maximum")) -> ()  [unwired: 2 in, 2 out]
                n191 = local write "Slider"(w301) -> ()
              }
            }
            n192 = property on="On/Off" class="Bool (strict)"("Visible"=FALSE) -> ()  [unwired: 2 in, 2 out]
            n193 = property on="Motor" class="Clust (strict)"("Visible"=FALSE) -> ()  [unwired: 2 in, 2 out]
          }
        }
      }
      event "Test Name": Mouse Enter {
        # "Populate the ring with the list of tests"
        n194 = event-data() -> ()  [unwired: 1 in, 1 out]
        n195 = call <vilib>:"NT Read String Array.vi"("Name"="TestMode/TestList") -> ("String Array"=w309:string[])  [unwired: 9 in, 1 out]
        n196 = Build Array (concatenate)("Select the test to run...", w309) -> (w308:string[])
        n197 = property on="Test Name" class="Ring (strict)"("Strings []"=w308) -> ()  [unwired: 2 in, 2 out]
      }
      event "Test Name": Value Change {
        w311 = FALSE ("Visible")
        # "Tell the robot the test name to run"
        n198 = event-data() -> ("NewVal"=w315:u16)  [unwired: 1 in]
        n199 = property on="Test Name" class="Ring (strict)"() -> ("Strings []"=w316:string[])  [unwired: 2 in, 2 out]
        n200 = property on="Ring" class="Ring (strict)"("Visible"=w311) -> ()  [unwired: 2 in, 2 out]
        n201 = property on="Motor" class="Clust (strict)"("Visible"=w311) -> ()  [unwired: 2 in, 2 out]
        n202 = property on="Slider" class="Slide (strict)"("Visible"=w311) -> ()  [unwired: 2 in, 2 out]
        n203 = property on="On/Off" class="Bool (strict)"("Visible"=w311) -> ()  [unwired: 2 in, 2 out]
        n204 = property on="Rev/Fwd" class="Clust (strict)"("Visible"=w311) -> ()  [unwired: 2 in, 2 out]
        n205 = local write "Progress"(T4 {"Test Progress"=0, "Test Progress Text"=""} ("Progress")) -> ()
        n206 = property on="Progress" class="Clust (strict)"("Visible"=TRUE) -> ()  [unwired: 2 in, 2 out]
        n207 = Index Array(array=w316, index=w315) -> (element=w314:string)
        n208 = call <vilib>:"NT Write String.vi"("String"=w314, "Name"="TestMode/TestName") -> ()  [unwired: 9 in, 1 out]
      }
      event "Listbox": Double Click {
        n209 = event-data() -> ("PlatMods.Shift"=w319:bool, "Row"=w321:i32)  [unwired: 1 in]
        n210 = case shown="False" w319 {
          tunnel: w321 -> [w325 _]
          tunnel: 1 -> [w324 _]
          frame False {
            n211 = property on="Listbox" class="LstBox (strict)"() -> ("Item Symbols"=w323:i32[])  [unwired: 2 in, 2 out]
            n212 = Replace Array Subset(array=w323, new element=w324, index=w325) -> (w322:i32[])
            n213 = property on="Listbox" class="LstBox (strict)"("Item Symbols"=w322) -> ()  [unwired: 2 in, 2 out]
          }
          frame True {
            w326 = 0 ("Top Row")
            n214 = property on="Listbox" class="LstBox (strict)"() -> ("Number of Rows"=w328:u32)  [unwired: 2 in, 2 out]
            n215 = Initialize Array(0, w328) -> (w327:i32[])
            n216 = property on="Listbox" class="LstBox (strict)"("Top Row"=w326, "Value"=w326, "Item Symbols"=w327) -> ()  [unwired: 2 in, 2 out]
          }
        }
      }
      event "Listbox": Key Down {
        n217 = event-data() -> ("VKey"=w332:T17)  [unwired: 1 in]
        n218 = case shown="\"Left\", \"Right\"" w332 {
          selector: w332 -> [w337 _]
          tunnel: eventvkey."Left" ("VKey") -> [w335 _]
          frame "Left", "Right" {
            n219 = Equal?(x=w335, y=w337) -> (x = y?=w336:bool)
            n220 = Select(t=0, s=w336, f=1) -> (s? t:f=w338:i32)
            n221 = property on="Listbox" class="LstBox (strict)"() -> ("Item Symbols"=w341:i32[])  [unwired: 2 in, 2 out]
            n222 = Replace Array Subset(array=w341, new element=w338, index="Listbox") -> (w340:i32[])
            n223 = property on="Listbox" class="LstBox (strict)"("Item Symbols"=w340) -> ()  [unwired: 2 in, 2 out]
          }
          frame Default {
          }
        }
      }
      event "DB Camera Config": Value Change {
        n224 = event-data() -> ("NewVal"=w345:bool)  [unwired: 1 in]
        n225 = case shown="False" w345 {
          tunnel: w344 -> [w354 _]
          tunnel: [w347 w365] -> w343
          tunnel: w342 -> [w346 w365]
          frame False {
            w361 = "Camera"
            w364 = FALSE ("Visible")
            n226 = property on="Camera Settings" class="Clust (strict)"("Visible"=w364) -> ()  [unwired: 2 in, 2 out]
            n227 = local write "DB Camera Config"(w364) -> ()
            n228 = local read "Camera Settings"() -> (w353:T2)
            n229 = Index Array(array=w354) -> (element=w357:cluster{string[]})  [unwired: 1 in]
            n230 = Unbundle(w357) -> (w356:string[])
            n231 = Unbundle(w353) -> ("Frate Rate"=w352:i32, "Compression"=w351:i32, "Size"=w355:u16)
            n232 = Index Array(array=w356, index=w355) -> (element=w350:string)
            n233 = call-poly <vilib>:"Write Key.vi"("section"=w361, "value"=w350, "key"="Size", "refnum"=w346) -> ("refnum out"=w363:T16)  [unwired: 2 in, 5 out]
            n234 = call-poly <vilib>:"Write Key.vi"("section"=w361, "value"=w352, "key"="FrameRate", "refnum"=w363) -> ("refnum out"=w362:T16)  [unwired: 1 in, 6 out]
            n235 = call-poly <vilib>:"Write Key.vi"("section"=w361, "value"=w351, "key"="Compression", "refnum"=w362) -> ("refnum out"=w348:T16)  [unwired: 1 in, 6 out]
            n236 = call <vilib>:"Close Config Data.vi"("refnum"=w348) -> ("file path"=w349:path)  [unwired: 2 in, 8 out]
            n237 = call <vilib>:"Open Config Data.vi"("configuration file path"=w349) -> ("refnum"=w347:T16)  [unwired: 8 in, 2 out]
          }
          frame True {
            n238 = property on="Camera Settings" class="Clust (strict)"("Visible"=TRUE) -> ()  [unwired: 2 in, 2 out]
          }
        }
      }
      event "Camera Settings": Value Change {
        n239 = event-data() -> ("NewVal"=w378:T2)  [unwired: 1 in]
        n240 = Index Array(array=w374) -> (element=w373:cluster{string[]})  [unwired: 1 in]
        n241 = Unbundle(w373) -> (w372:string[])
        n242 = Unbundle(w378) -> ("Frate Rate"=w369:i32, "Compression"=w368:i32, "Size"=w371:u16)
        n243 = Index Array(array=w372, index=w371) -> (element=w370:string)
        n244 = Format Into String(format string="%s   %dfps   %d%%", w370, w369, w368) -> (resulting string=w375:string)  [unwired: 2 in, 1 out]
        n245 = Build Array(w375) -> (w376:string[])
        n246 = property on="DB Camera Config" class="Bool (strict)"("Strings [4]"=w376) -> ()  [unwired: 2 in, 2 out]
      }
      event "Motor.Enable": Value Change {
        n247 = event-data() -> ("NewVal"=w384:bool)  [unwired: 1 in]
        n248 = Unbundle("Motor") -> ("Value"=w383:dbl)  [unwired: 1 out]
        n249 = Select(t=w383, s=w384, f=0.0) -> (s? t:f=w381:dbl)
        n250 = call <vilib>:"NT Write Number.vi"("Numeric"=w381, "Name"=w380) -> ()  [unwired: 9 in, 1 out]
      }
      event "Slider": Value Change {
        n251 = event-data() -> ("NewVal"=w387:dbl)  [unwired: 1 in]
        n252 = call <vilib>:"NT Write Number.vi"("Numeric"=w387, "Name"=w388) -> ()  [unwired: 9 in, 1 out]
      }
      event "On/Off": Value Change {
        n253 = event-data() -> ("NewVal"=w392:bool)  [unwired: 1 in]
        n254 = Boolean To (0,1)(Boolean=w392) -> (0, 1=w391:i16)
        n255 = call <vilib>:"NT Write Number.vi"("Numeric"=w391, "Name"=w390) -> ()  [unwired: 9 in, 1 out]
      }
      event "Rev/Fwd": Value Change {
        n256 = event-data() -> ("NewVal.Forward"=w400:bool, "NewVal.Reverse"=w399:bool)  [unwired: 1 in]
        n257 = Boolean To (0,1)(Boolean=w399) -> (0, 1=w398:i16)
        n258 = Boolean To (0,1)(Boolean=w400) -> (0, 1=w396:i16)
        n259 = Negate(x=w398) -> (-x=w397:i16)
        n260 = Add(x=w396, y=w397) -> (x+y=w395:i16)
        n261 = call <vilib>:"NT Write Number.vi"("Numeric"=w395, "Name"=w394) -> ()  [unwired: 9 in, 1 out]
      }
      event "Ring": Value Change {
        n262 = event-data() -> ("NewVal"=w404:u16)  [unwired: 1 in]
        n263 = property on="Ring" class="Ring (strict)"() -> ("Strings []"=w405:string[])  [unwired: 2 in, 2 out]
        n264 = Index Array(array=w405, index=w404) -> (element=w403:string)
        n265 = call <vilib>:"NT Write String.vi"("String"=w403, "Name"=w402) -> ()  [unwired: 9 in, 1 out]
      }
    }
  }
  n266 = property on="Camera Settings" class="Clust (strict)"("Val(Sgnl)"=w4) -> ()  [unwired: 2 in, 2 out]
